vi "set_do.vi"(8 "error in":errorcluster, 9 "on/off":bool, 10 "Digital output":u16 max=3 step=1, 11 "Modbus Master in":refnum<class "Modbus Master.lvclass">) -> (0 "error out":errorcluster, 3 "Modbus Master out":refnum<class "Modbus Master.lvclass">)   [LabVIEW 2018, in "ICP xET-7017.lvlib"]
uses:
  ICP xET-7017.lvlib
  <vilib>/NI/Modbus Library/API/Master/Modbus Master.lvclass
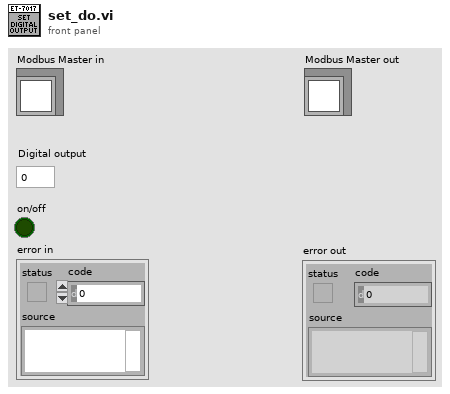
[diagram p1: front panel]
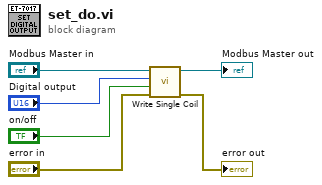
[diagram p0: block diagram]
diagram:
  n1 = call-dynamic "Write Single Coil.vi"("error in"="error in", "coil to write"="on/off", "address"="Digital output", "Modbus master in"="Modbus Master in") -> ("error out"=→"error out":errorcluster, "Modbus master out"=→"Modbus Master out":refnum<class "Modbus Master.lvclass">)  [unwired: 6 in]
